vi "load_udc_table.vi"(1 "name or relative path":string="udc3200_table.txt") -> (0 "UDC Table":string[][](array[string]))   [LabVIEW 2011]
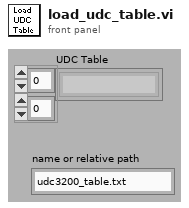
[diagram p1: front panel]
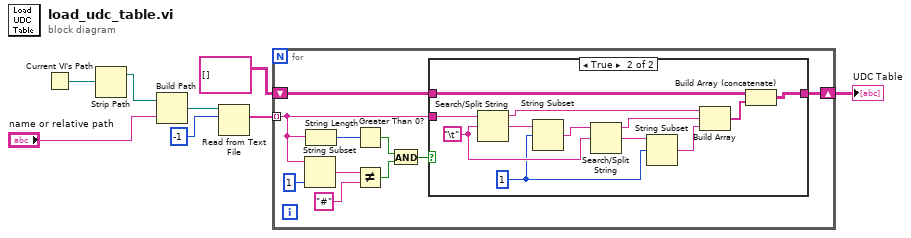
[diagram p0: block diagram]
diagram:
  n1 = Current VI's Path() -> (path=w6:path)
  n2 = Strip Path(path=w6) -> (stripped path=w5:path)  [unwired: 1 out]
  n3 = Build Path(base path=w5, name or relative path="name or relative path") -> (appended path=w7:path)
  n4 = Read from Text File(file (use dialog)=w7, count=-1) -> (text=w4:string[])  [unwired: 1 in, 4 out]
  n5 = for {
    tunnel: w4 -> [w13] mode=indexing
    shift-right: [w15] -> w2
    shift-left: string[][] [] -> [w16]
    n6 = String Subset(string=w13, length (rest)=1 ("length (rest)")) -> (substring=w14:string)  [unwired: 1 out]
    n7 = String Length(string=w13) -> (length=w12:i32)
    n8 = Greater Than 0?(x=w12) -> (x > 0?=w10:bool)
    n9 = Not Equal?(x=w14, y="#") -> (x != y?=w9:bool)
    n10 = And(x=w10, y=w9) -> (x .and. y?=w11:bool)
    n11 = case shown="True" w11 {
      tunnel: w13 -> [_ w23]
      tunnel: w16 -> [w19 w20]
      tunnel: [w19 w21] -> w15
      frame False {
      }
      frame True {
        w27 = 1 ("offset (0)")
        w31 = "\t"
        n12 = Search/Split String(string=w23, search string/char (-)=w31) -> (substring before match=w24:string, match + rest of string=w25:string)  [unwired: 2 out]
        n13 = String Subset(string=w25, offset (0)=w27) -> (substring=w26:string)  [unwired: 1 out]
        n14 = Search/Split String(string=w26, search string/char (-)=w31) -> (substring before match=w30:string, match + rest of string=w29:string)  [unwired: 2 out]
        n15 = String Subset(string=w29, offset (0)=w27) -> (substring=w28:string)  [unwired: 1 out]
        n16 = Build Array(w24, w30, w28) -> (w22:string[])
        n17 = Build Array (concatenate)(w20, w22) -> (w21:string[][])
      }
    }
  }
  "UDC Table" <- w2
